vi "PolynomialFit.vi"() -> ()   [LabVIEW 2015]
uses:
  <vilib>/imath/engines/lvmath2/RunTimeEngine/BuiltInFunctions/polyfit/NIMS_[2o]_polyfit.vi
  <vilib>/imath/engines/lvmath2/RunTimeEngine/ErrorHandling/NIMS_Error From Error Code.vi
  <vilib>/imath/engines/lvmath2/RunTimeEngine/IndexRead/NIMS V(S).vi
  <instcachedir>/0/NIMS V(S)_0488751826AF41519A22953C041130DC.lvgen/NIMS V(S)_0488751826AF41519A22953C041130DC_000.vi
  <vilib>/imathl/engines/lvmath/Functions/Error Handling/Create Error.vi
  <vilib>/imath/engines/lvmath2/RunTimeEngine/NodeEndStatement/NIMS_NodeEndStatement_Output.vi
  <instcachedir>/0/NIMS_NodeEndStatement_Output_53EC0D466D134D7ABD903AC30B43404B.lvgen/NIMS_NodeEndStatement_Output_53EC0D466D134D7ABD903AC30B43404B_005.vi
  <instcachedir>/0/NIMS_NodeEndStatement_Output_53EC0D466D134D7ABD903AC30B43404B.lvgen/NIMS_NodeEndStatement_Output_53EC0D466D134D7ABD903AC30B43404B_001.vi
  <vilib>/imath/engines/lvmath2/RunTimeEngine/ErrorHandling/NIMS_Finalize Error.vi
  <vilib>/Analysis/polynomials.llb/Polynomial Plot (Samples).vi
  <vilib>/Analysis/NI_AALPro.lvlib
panel:
  out "XY Graph":cluster{"x":dbl[], "P(A)":dbl[]}[](graph)
  out "a2":dbl
  out "a1":dbl
  out "a0":dbl
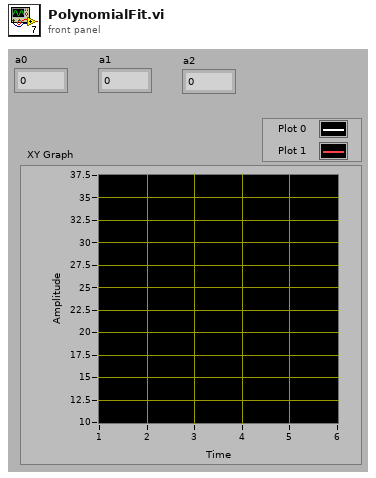
[diagram p1: front panel]
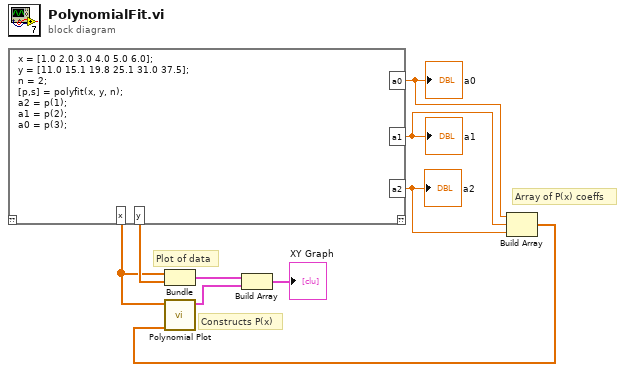
[diagram p0: block diagram]
diagram:
  # "Plot of data"
  # "Constructs P(x)"
  # "Array of P(x) coeffs"
  n1 = mathscript code="x = [1.0 2.0 3.0 4.0 5.0 6.0];\ny = [11.0 15.1 19.8 25.1 31.0 37.5];\nn = 2;\n[p,s] = polyfit(x, y, n);\na2 = p(1);\na1 = p(2);\na0 = p(3);"() -> ("a0"=w7:dbl, "a1"=w6:dbl, "a2"=w5:dbl, "x"=w8:dbl[], "y"=w9:dbl[])  [unwired: 1 in, 1 out]
  "a0" <- w7
  "a1" <- w6
  "a2" <- w5
  n2 = Bundle("x"=w8, "y"=w9) -> (w3:cluster{"x":dbl[], "y":dbl[]})  [unwired: 1 in]
  n3 = Build Array(w7, w6, w5) -> (w4:dbl[])
  n4 = call-poly <vilib>:"Polynomial Plot.vi"("P(x)"=w4, "X"=w8) -> ("polynomial plot"=w2:cluster{dbl[], "P(A)":dbl[]})  [unwired: 8 in, 1 out]
  n5 = Build Array(w3, w2) -> (→"XY Graph":cluster{"x":dbl[], "P(A)":dbl[]}[])
